vi "port Handler.vi"(8 "error in (no error)":errorcluster, 11 "port_name":string) -> (0 "error out":errorcluster, 3 "function return":i32)   [LabVIEW 2018, in "labview.lvlib"]
doc: "WINDECLSPEC int portHandler (const char *port_name);"
uses:
  labview.lvlib
  dxl_x86_c.dll
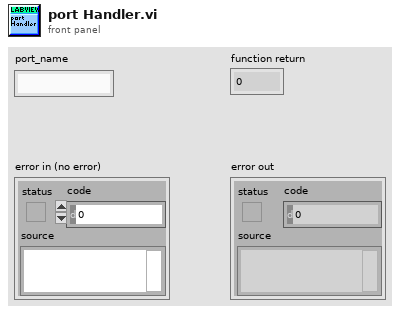
[diagram p1: front panel]
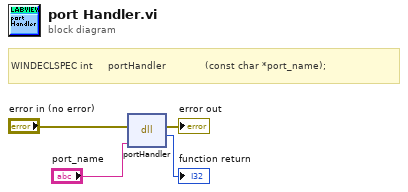
[diagram p0: block diagram]
diagram:
  # "WINDECLSPEC int     portHandler             (const char *port_name);"
  n1 = dll-call lib="C:/Users/joaos/OneDrive/Documents/[PhD]/Project Omnidirectional Vehicle/Vanes/LabView_code/joaoandthethreestands/DynamixelSDK-3.7.31/labview/new_compilation/dxl_x86_c.*" fn="portHandler"(error in="error in (no error)", "port_name"="port_name") -> (error out=→"error out":errorcluster, →"function return":i32)  [unwired: 3 in, 1 out]
